vi "LabVIEW Object to VCluster.vi"(8 "error in (no error)":errorcluster, 10 "LabVIEW Object":variant) -> (0 "error out":errorcluster, 2 "VCluster":variant)   [LabVIEW 2020, in "openg_variant.lvlib"]
doc: "Returns the elements of a cluster as an array of variant data."
uses:
  openg_variant.lvlib
  LabVIEW Object/Reflection/getObjectPrivateData.vi
  LabVIEW Object/Reflection/extractObjectPrivateDataValues.vi
  <vilib>/Utility/LVClass/Get LV Class Name.vi
  LabVIEW Object/Reflection/reflectionPool.vi
  Cluster to Array of VData.vi
  Set Data Name.vi
  Array of VData to VCluster.vi
panel:
  # "[OpenG VI Tags] ***Do Not Remove***"
  # "EXPERIMENTAL"
  # "LabVIEW Object to VCluster.vi\n\nReturns the elements of a cluster as an array of variant data.\n\nPlease visit http://www.OpenG.org to learn about the\nOpen Source LabVIEW software movement.\n\nNOTICE -- YOU MUST LEAVE THIS NOTICE IN PLACE.  PER THE TERMS OF THE LICENSE BELOW, YOU MAY SUBLICENSE THIS SOFTWARE \nIN ANY WAY THAT DOES NOT CONFLICT WITH THIS LICENSE.\n\n### BSD License (http://www.opensource.org/licenses/bsd-license.php) Begin ###\n \nCopyright (c) 2002, Jean-Pierre Drolet <drolet_jp@hotmail.com>\nCopyright (c) 2002-2006, Jim Kring <jim@jimkring.com>\n\nAll rights reserved.\n\nRedistribution and use in source and binary forms, with or without modification, are permitted provided that the following conditions are met:\n\n    * Redistributions of source code must retain the above copyright notice, this list of conditions and the following disclaimer.\n    * Redistributions in binary form must reproduce the above copyright notice, this list of conditions and the following disclaimer in the \n       documentation and/or other materials provided with the distribution.\n    * Neither the name of SciWare, James Kring, Inc., nor the names of its contributors may be used to endorse or promote products derived \n       from this software without specific prior written permission.\n\nTHIS SOFTWARE IS PROVIDED BY THE COPYRIGHT HOLDERS AND CONTRIBUTORS \"AS IS\" AND ANY EXPRESS OR IMPLIED WARRANTIES, \nINCLUDING, BUT NOT LIMITED TO, THE IMPLIED WARRANTIES OF MERCHANTABILITY AND FITNESS FOR A PARTICULAR PURPOSE ARE \nDISCLAIMED. IN NO EVENT SHALL THE COPYRIGHT OWNER OR CONTRIBUTORS BE LIABLE FOR ANY DIRECT, INDIRECT, INCIDENTAL,\n SPECIAL, EXEMPLARY, OR CONSEQUENTIAL DAMAGES (INCLUDING, BUT NOT LIMITED TO, PROCUREMENT OF SUBSTITUTE GOODS OR \nSERVICES; LOSS OF USE, DATA, OR PROFITS; OR BUSINESS INTERRUPTION) HOWEVER CAUSED AND ON ANY THEORY OF LIABILITY, \nWHETHER IN CONTRACT, STRICT LIABILITY, OR TORT (INCLUDING NEGLIGENCE OR OTHERWISE) ARISING IN ANY WAY OUT OF THE USE \nOF THIS SOFTWARE, EVEN IF ADVISED OF THE POSSIBILITY OF SUCH DAMAGE.\n\n### BSD License End ###"
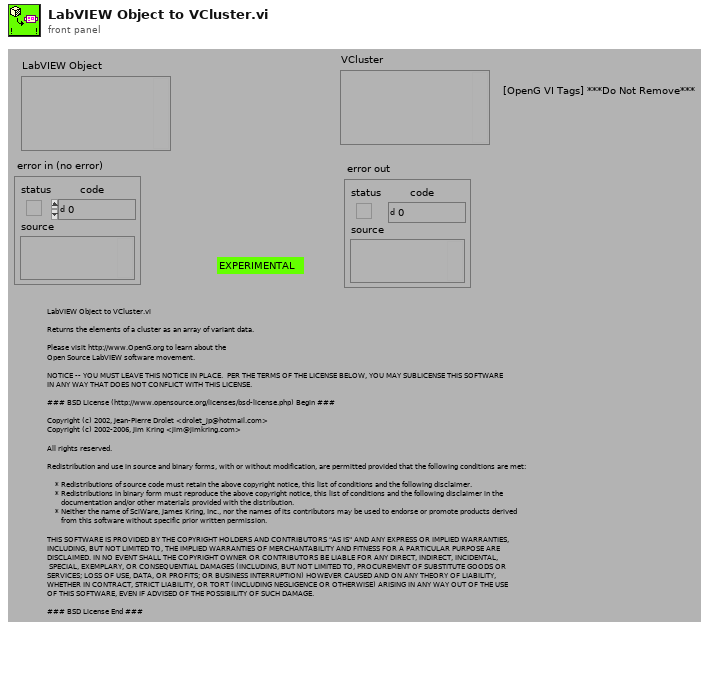
[diagram p1: front panel]
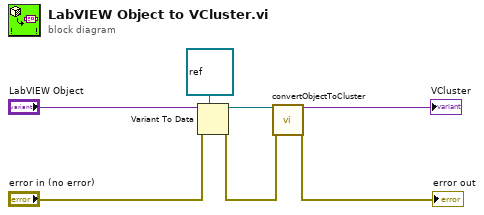
[diagram p0: block diagram]
diagram:
  n1 = Variant To Data(error in="error in (no error)", type=refnum<class> refnum ("objectType"), Variant="LabVIEW Object") -> (data=w4:refnum<class>, error out=w3:errorcluster)
  n2 = call "convertObjectToCluster.vi"("LabVIEW Object in"=w4, "error in (no error)"=w3) -> ("VCluster"=→"VCluster":variant, "error out"=→"error out":errorcluster)  [unwired: 16 in]
